vi "AWS IoT Button - Send SQS Message.vi"() -> ()   [LabVIEW 2015]
doc: "Demonstrates how to programmatically send AWS IoT Button data to an SQS queue."
uses:
  Core/HTTP Request/Region.ctl
  IoT/Topic Rule.ctl
  IoT/CloudWatch Alarm.ctl
  IoT/CloudWatch Metric.ctl
  IoT/DynamoDB.ctl
  IoT/DynamoDBv2.ctl
  IoT/Elasticsearch.ctl
  IoT/Firehose.ctl
  IoT/Kinesis.ctl
  IoT/Lambda.ctl
  IoT/Republish.ctl
  IoT/S3.ctl
  IoT/SNS.ctl
  IoT/SQS.ctl
  Core/HTTP Request/AWS Credentials.ctl
  SQS/Queue/Queue.lvclass/Queue.ctl
  SQS/Queue/Read URL.vi
  IoT/IoT Session/IoT Session.lvclass
  IoT/NI_AWS_IoT.lvlib
  SQS/Queue/Queue.lvclass
  Core/HTTP Request/HTTP Request.lvclass
panel:
  out "Ready":bool
  in  "SQS Queue":string
  in  "AWS IoT Button Serial Number":string
  in  "Region":T1
  in  "Secret Key":string
  in  "Access Key":string
  in  "Stop":bool
  out "Messages":string[][](table)
  # "Overview: Demonstrates how to programmatically send AWS IoT Button data to an SQS queue.\nRequirements: NI Cloud Toolkit for AWS, a configured AWS IoT Button, and a registered Amazon AWS account\nInstructions:\n1. Specify the Access Key and Secret Key for your AWS account. You can create an account at http://aws.amazon.com.\n2. Make sure you already have an AWS IoT Button configured in the AWS IoT Management Console on the amazon website.\n3. Specify the Region under which your AWS IoT Button is configured.\n4. Specify the AWS IoT Button Serial Number.\n5. Specify the SQS Queue where you want to send the AWS IoT Button data. Note: This queue must already exist, and it must be in the same region as the AWS IoT Button.\n6. Run the VI.\n7. After the Ready LED turns on, click the AWS IoT Button. After the green light appears on the button, you should see a new entry in the Messages table below."
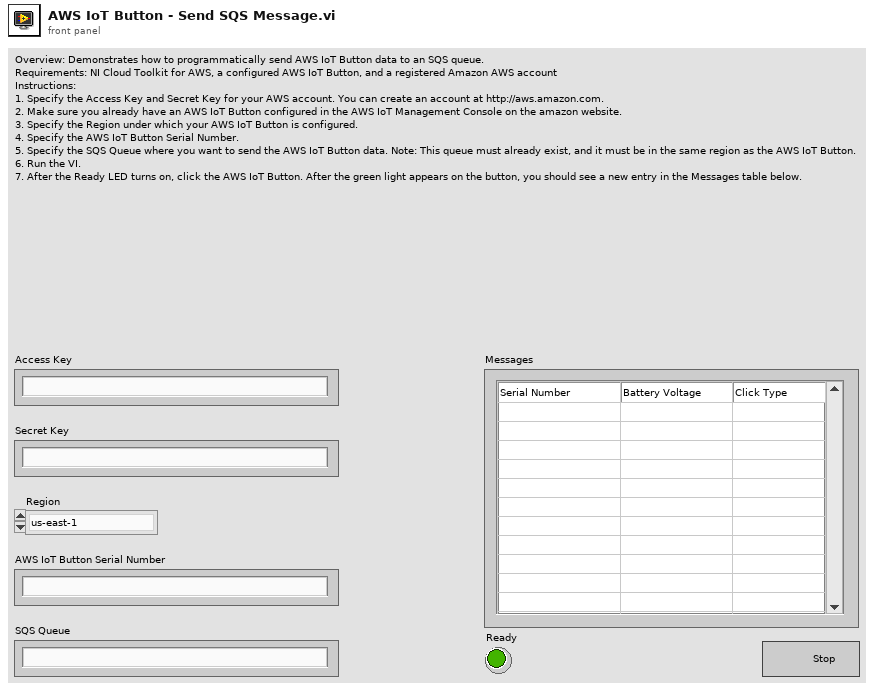
[diagram p1: front panel]
types:
  T1 = typedef "NI_AWS_Core.lvlib/HTTP Request.lvclass/Region.ctl" = enum16{"us-east-1", "us-east-2", "us-west-1", "us-west-2", "ap-northeast-1", "ap-northeast-2", "ap-southeast-1", "ap-southeast-2", "ca-central-1", "eu-central-1", "eu-west-1", "eu-west-2", "sa-east-1"}
  T2 = typedef "NI_AWS_Core.lvlib/HTTP Request.lvclass/AWS Credentials.ctl" = cluster{"Access Key":string, "Secret Key":string}
  T3 = typedef "NI_AWS_IoT.lvlib/SQS.ctl" = cluster{"Queue URL":string, "Role ARN":string, "Use Base 64":bool}
  T4 = typedef "NI_AWS_IoT.lvlib/Topic Rule.ctl" = cluster{"CloudWatch Alarm":T5[], "CloudWatch Metric":T6[], "DynamoDB":T7[], "DynamoDBv2":T8[], "Elasticsearch":T9[], "Firehose":T10[], "Kinesis":T11[], "Lambda":T12[], "Republish":T13[], "S3":T14[], "SNS":T15[], "SQS":T3[], "AWS IoT SQL Version":string, "Description":string, "Created At":u64, "Incoming Schema ARN":string, "Outgoing Schema ARN":string, "Rule Disabled":bool, "Rule Name":string, "SQL":string, "Rule ARN":string}
  T5 = typedef "NI_AWS_IoT.lvlib/CloudWatch Alarm.ctl" = cluster{"Alarm Name":string, "Role ARN":string, "State Reason":string, "State Value":string}
  T6 = typedef "NI_AWS_IoT.lvlib/CloudWatch Metric.ctl" = cluster{"Metric Name":string, "Metric Namespace":string, "Metric Timestamp":string, "Metric Unit":string, "Metric Value":string, "Role ARN":string}
  T7 = typedef "NI_AWS_IoT.lvlib/DynamoDB.ctl" = cluster{"Hash Key Field":string, "Hash Key Type":string, "Hash Key Value":string, "Operation":string, "Payload Field":string, "Range Key Field":string, "Range Key Type":string, "Range Key Value":string, "Role ARN":string, "Table Name":string}
  T8 = typedef "NI_AWS_IoT.lvlib/DynamoDBv2.ctl" = cluster{"Role ARN":string, "Table Name":string}
  T9 = typedef "NI_AWS_IoT.lvlib/Elasticsearch.ctl" = cluster{"Endpoint":string, "ID":string, "Index":string, "Role ARN":string, "Type":string}
  T10 = typedef "NI_AWS_IoT.lvlib/Firehose.ctl" = cluster{"Delivery Stream Name":string, "Role ARN":string, "Separator":string}
  T11 = typedef "NI_AWS_IoT.lvlib/Kinesis.ctl" = cluster{"Partition Key":string, "Role ARN":string, "Stream Name":string}
  T12 = typedef "NI_AWS_IoT.lvlib/Lambda.ctl" = cluster{"Function ARN":string}
  T13 = typedef "NI_AWS_IoT.lvlib/Republish.ctl" = cluster{"Role ARN":string, "Topic":string}
  T14 = typedef "NI_AWS_IoT.lvlib/S3.ctl" = cluster{"Bucket Name":string, "Canned ACL":string, "Key":string, "Role ARN":string}
  T15 = typedef "NI_AWS_IoT.lvlib/SNS.ctl" = cluster{"Message Format":string, "Role ARN":string, "Target ARN":string}
  T16 = typedef "NI_AWS_SQS.lvlib/Queue.lvclass/Message.ctl" = cluster{"Body":string, "MD5 of Body":string, "ID":string, "Receipt Handle":string, "Native Attributes":T17[], "Custom Attributes":T19[], "MD5 of Custom Attributes":string}
  T17 = typedef "NI_AWS_SQS.lvlib/Queue.lvclass/Message Attribute Value Pair.ctl" = cluster{"Attribute":T18, "Value":string}
  T18 = typedef "NI_AWS_SQS.lvlib/Queue.lvclass/Message Attribute.ctl" = enum16{"SenderId", "SentTimestamp", "ApproximateReceiveCount", "ApproximateFirstReceiveTimestamp"}
  T19 = typedef "NI_AWS_SQS.lvlib/Queue.lvclass/Custom Attribute.ctl" = cluster{"Name":string, "Type":T20, "Value":string}
  T20 = typedef "NI_AWS_SQS.lvlib/Queue.lvclass/Custom Attribute Type.ctl" = enum16{"String", "Number", "Binary"}
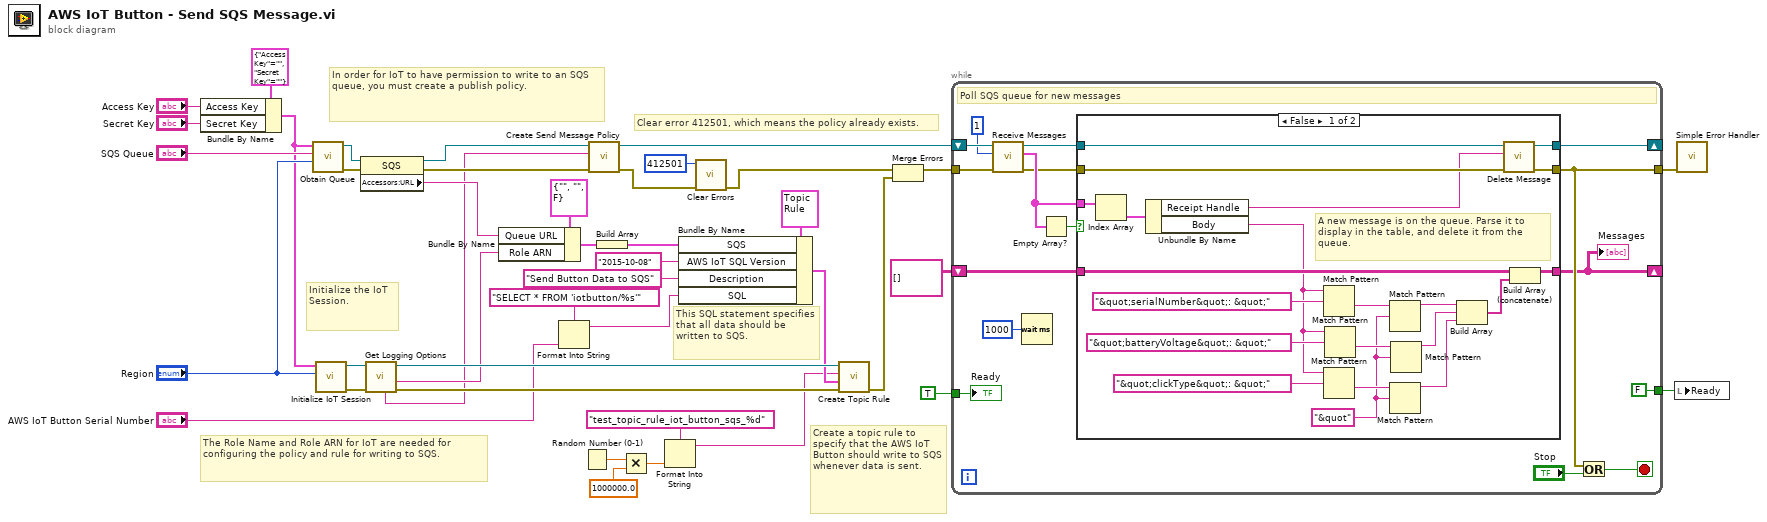
[diagram p0: block diagram]
diagram:
  # "This SQL statement specifies that all data should be written to SQS."
  # "In order for IoT to have permission to write to an SQS queue, you must create a publish policy."
  # "Clear error 412501, which means the policy already exists."
  # "Create a topic rule to specify that the AWS IoT Button should write to SQS whenever data is sent."
  # "The Role Name and Role ARN for IoT are needed for configuring the policy and rule for writing to SQS."
  # "Initialize the IoT Session."
  n1 = Bundle By Name(cluster=T2 {"Access Key"="", "Secret Key"=""} ("AWS Credentials"), "Access Key"="Access Key", "Secret Key"="Secret Key") -> (w10:T2)
  n2 = call "Obtain Queue.vi"("Region"="Region", "Name"="SQS Queue", "AWS Credentials"=w10) -> ("error out"=w39:errorcluster, "SQS"=w38:refnum<class "Queue.lvclass">)  [unwired: 7 in]
  n3 = call "Initialize IoT Session.vi"("Region"="Region", "AWS Credentials"=w10) -> ("error out"=w42:errorcluster, "IoT Session"=w35:refnum<class "IoT Session.lvclass">)  [unwired: 8 in]
  n4 = property class="SQS"(reference=w38, error in=w39) -> (reference out=w16:refnum<class "Queue.lvclass">, error out=w23:errorcluster, "Accessors:URL"=w37:string)
  n5 = call "Get Logging Options.vi"("error in (no error)"=w42, "IoT Session in"=w35) -> ("error out"=w36:errorcluster, "Role ARN"=w33:string, "IoT Session out"=w34:refnum<class "IoT Session.lvclass">, "Role Name"=w14:string)  [unwired: 5 in, 1 out]
  n6 = Bundle By Name(cluster=T3 {"Queue URL"="", "Role ARN"="", "Use Base 64"=FALSE} ("SQS"), "Queue URL"=w37, "Role ARN"=w33) -> (w32:T3)
  n7 = Format Into String(format string="SELECT * FROM 'iotbutton/%s'", "AWS IoT Button Serial Number") -> (resulting string=w26:string)  [unwired: 2 in, 1 out]
  n8 = Random Number (0-1)() -> (number: 0 to 1=w25:dbl)
  n9 = call "Create Send Message Policy.vi"("error in (no error)"=w23, "Role Name"=w14, "SQS in"=w16) -> ("error out"=w2:errorcluster, "SQS out"=w15:refnum<class "Queue.lvclass">)  [unwired: 7 in]
  n10 = Build Array(w32) -> (w31:T3[])
  n11 = Multiply(x=w25, y=1000000.0) -> (x*y=w18:dbl)
  n12 = Format Into String(format string="test_topic_rule_iot_button_sqs_%d" ("Name"), w18) -> (resulting string=w17:string)  [unwired: 2 in, 1 out]
  n13 = Bundle By Name(cluster=T4 {"CloudWatch Alarm"=[], "CloudWatch Metric"=[], "DynamoDB"=[], "DynamoDBv2"=[], "Elasticsearch"=[], "Firehose"=[], "Kinesis"=[], "Lambda"=[], "Republish"=[], "S3"=[], "SNS"=[], "SQS"=[], "AWS IoT SQL Version"="", "Description"="", "Created At"=0, "Incoming Schema ARN"="", "Outgoing Schema ARN"="", "Rule Disabled"=FALSE, "Rule Name"="", "SQL"="", "Rule ARN"=""} ("Topic Rule"), "SQS"=w31, "AWS IoT SQL Version"="2015-10-08", "Description"="Send Button Data to SQS", "SQL"=w26) -> (w28:T4)
  n14 = call <vilib>:"Clear Errors.vi"("error in (no error)"=w2, "specific error code to clear (0: all)"=412501) -> ("error out"=w1:errorcluster)  [unwired: 4 in, 1 out]
  n15 = call "Create Topic Rule.vi"("error in (no error)"=w36, "Topic Rule"=w28, "Rule Name"=w17, "IoT Session in"=w34) -> ("error out"=w22:errorcluster)  [unwired: 6 in, 1 out]
  n16 = Merge Errors(w1, w22) -> (w21:errorcluster)
  n17 = while {
    tunnel: w21 -> [w58]
    shift-right: [w48] -> _
    shift-left: w15 -> [w57]
    tunnel: [w47] -> w6
    shift-right: [w45] -> _
    shift-left: string[][] [] ("Messages") -> [w46]
    tunnel: TRUE -> [w44]
    tunnel: [FALSE] -> w4
    stop <- w54 stop-if-true
    # "Poll SQS queue for new messages"
    n18 = call "Receive Messages.vi"("error in (no error)"=w58, "Max Number of Messages"=1, "SQS in"=w57) -> ("error out"=w50:errorcluster, "Messages"=w51:T16[], "SQS out"=w49:refnum<class "Queue.lvclass">)  [unwired: 6 in]
    n19 = Wait (ms)(milliseconds to wait=u32 1000) -> ()  [unwired: 1 out]
    n20 = Empty Array?(array=w51) -> (empty?=w52:bool)
    n21 = case shown="False" w52 {
      tunnel: w51 -> [w79 _]
      tunnel: w50 -> [w74 w81]
      tunnel: w49 -> [w77 w82]
      tunnel: [w76 w82] -> w48
      tunnel: [w75 w81] -> w47
      tunnel: w46 -> [w72 w80]
      tunnel: [w71 w80] -> w45
      frame False {
        w59 = "&quot"
        # "A new message is on the queue. Parse it to display in the table, and delete it from the queue."
        n22 = Index Array(array=w79) -> (element=w78:T16)  [unwired: 1 in]
        n23 = Unbundle By Name(w78) -> ("Receipt Handle"=w73:string, "Body"=w62:string)
        n24 = Match Pattern(string=w62, regular expression="&quot;serialNumber&quot;: &quot;") -> (after substring=w68:string)  [unwired: 1 in, 3 out]
        n25 = Match Pattern(string=w62, regular expression="&quot;clickType&quot;: &quot;") -> (after substring=w63:string)  [unwired: 1 in, 3 out]
        n26 = Match Pattern(string=w62, regular expression="&quot;batteryVoltage&quot;: &quot;") -> (after substring=w66:string)  [unwired: 1 in, 3 out]
        n27 = Match Pattern(string=w68, regular expression=w59) -> (before substring=w67:string)  [unwired: 1 in, 3 out]
        n28 = Match Pattern(string=w63, regular expression=w59) -> (before substring=w60:string)  [unwired: 1 in, 3 out]
        n29 = Match Pattern(string=w66, regular expression=w59) -> (before substring=w61:string)  [unwired: 1 in, 3 out]
        n30 = Build Array(w67, w61, w60) -> (w70:string[])
        n31 = call "Delete Message.vi"("error in (no error)"=w74, "Receipt Handle"=w73, "SQS in"=w77) -> ("error out"=w75:errorcluster, "SQS out"=w76:refnum<class "Queue.lvclass">)  [unwired: 7 in]
        n32 = Build Array (concatenate)(w72, w70) -> (w71:string[][])
      }
      frame True {
        # "No new messages on the queue."
      }
    }
    "Messages" <- w45
    n33 = Or(x=w47, y="Stop") -> (x .or. y?=w54:bool)
    "Ready" <- w44
  }
  n34 = local write "Ready"(w4) -> ()
  n35 = call <vilib>:"Simple Error Handler.vi"("error in (no error)"=w6) -> ()  [unwired: 4 in, 5 out]
